vi "Single PWM.vi"() -> ()   [LabVIEW 2020, in "CTI-Visa-Scratchpad.lvlib"]
uses:
  CTI-Visa-Scratchpad.lvlib
  CTI-Visa/CTI-Visa.lvlib
panel:
  out "Act. Freq":sgl format="%.4f"
  out "Act. Duty":sgl format="%_6f"
  in  "Frequency":sgl(slide) scale=10.0..500000.0
  in  "stop":bool
  in  "Port":refnum<visa-resource-name>="COM3"
  in  "Duty":sgl(slide) scale=0.0..1.0
  in  "Channel":i32
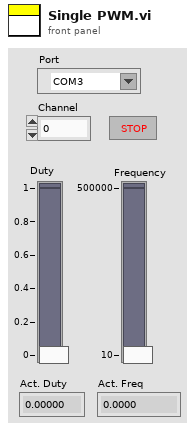
[diagram p1: front panel]
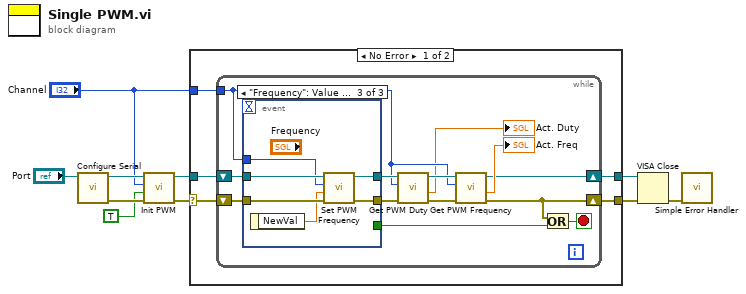
[diagram p0: block diagram]
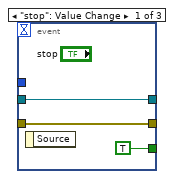
[diagram p2: hidden frame]
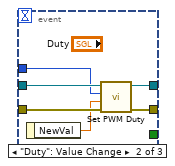
[diagram p3: hidden frame]
diagram:
  n1 = call "Configure Serial.vi"("VISA resource name in"="Port") -> ("error out"=w8:errorcluster, "VISA resource name"=w9:refnum<visa-resource-name>)  [unwired: 9 in]
  n2 = call "Init PWM.vi"("error in (no error)"=w8, "Enable (F)"=TRUE, "Channel"="Channel", "VISA resource name in"=w9) -> ("error out"=w7:errorcluster, "VISA resource name"=w6:refnum<visa-resource-name>)  [unwired: 6 in]
  n3 = case shown="No Error" w7 {
    selector: w7 -> [w14 w44]
    tunnel: w6 -> [w15 w45]
    tunnel: [w13 w45] -> w3
    tunnel: [w12 w44] -> w4
    tunnel: "Channel" -> [w11 _]
    frame No Error {
      n4 = while {
        shift-right: [w16] -> w13
        shift-left: w15 -> [w27]
        shift-right: [w17] -> w12
        shift-left: w14 -> [w26]
        tunnel: w11 -> [w21]
        stop <- w28 stop-if-true
        n5 = event shown="[2] \"Frequency\": Value Change" {
          selector: _ -> [_ _ _]
          dyn-events: _ -> [_ _ _]
          timeout: _ -> [_ _ _]
          tunnel: [w31 w33 w39] -> w24
          tunnel: w27 -> [w31 w37 w43]
          tunnel: [w30 w32 w38] -> w22
          tunnel: w26 -> [w30 w36 w42]
          tunnel: [TRUE _ _] -> w25
          tunnel: w21 -> [_ w34 w40]
          event "stop": Value Change {
            n6 = event-data() -> ()  [unwired: 1 in, 1 out]
          }
          event "Duty": Value Change {
            n7 = event-data() -> ("NewVal"=w35:sgl)  [unwired: 1 in]
            n8 = call "Set PWM Duty.vi"("error in (no error)"=w36, "Duty % (0-1)"=w35, "Channel"=w34, "VISA resource name in"=w37) -> ("error out"=w32:errorcluster, "VISA resource name"=w33:refnum<visa-resource-name>)  [unwired: 6 in]
          }
          event "Frequency": Value Change {
            n9 = event-data() -> ("NewVal"=w41:sgl)  [unwired: 1 in]
            n10 = call "Set PWM Frequency.vi"("error in (no error)"=w42, "Freq Hz"=w41, "Channel"=w40, "VISA resource name in"=w43) -> ("error out"=w38:errorcluster, "VISA resource name"=w39:refnum<visa-resource-name>)  [unwired: 6 in]
          }
        }
        n11 = call "Get PWM Duty.vi"("error in (no error)"=w22, "Channel"=w21, "VISA resource name in"=w24) -> ("error out"=w18:errorcluster, "Duty % (0-1)"=→"Act. Duty":sgl, "VISA resource name"=w23:refnum<visa-resource-name>)  [unwired: 6 in]
        n12 = call "Get PWM Frequency.vi"("error in (no error)"=w18, "Channel"=w21, "VISA resource name in"=w23) -> ("error out"=w17:errorcluster, "Freq Hz"=→"Act. Freq":sgl, "VISA resource name"=w16:refnum<visa-resource-name>)  [unwired: 6 in]
        n13 = Or(x=w17, y=w25) -> (x .or. y?=w28:bool)
      }
    }
    frame Error {
    }
  }
  n14 = VISA Close(VISA resource name=w3, error in (no error)=w4) -> (error out=w2:errorcluster)
  n15 = call <vilib>:"Simple Error Handler.vi"("error in (no error)"=w2) -> ()  [unwired: 4 in, 5 out]
